vi "Add Network Chassis.vi"(0 "SLSC Remote in":refnum<class "SLSC Remote.lvclass">, 1 "username":string, 2 "password":string, 5 "chassis IP address/hostname":string, 11 "error in (no error)":errorcluster, 12 "connect timeout (60 sec)":dbl=60.0) -> (4 "SLSC Remote out":refnum<class "SLSC Remote.lvclass">, 6 "chassis out":refnum<k21>, 15 "error out":errorcluster)   [LabVIEW 2015, in "SLSC Remote.lvclass"]
uses:
  SLSC Remote.lvclass
  <vilib>/NI/i3 JSON/JSON Generation/Create Value Files/Create Value - Object.vi
  <vilib>/NI/i3 JSON/JSON Generation/Add Object Parameter Files/Add Object Parameter - String.vi
  <vilib>/NI/i3 JSON/JSON Generation/Add Object Parameter Files/Add Object Parameter - Numeric.vi
  <vilib>/NI/NI JSONRPC Server Framework/Classes/Server/Format Client Request (Auto-Increment).vi
  <vilib>/httpClient/POSTBuffer.vi
  <vilib>/NI/i3 JSON/JSON Parsing/Get Object Parameter Files/Get Object Parameter - String.vi
  <vilib>/NI/NI JSONRPC Server Framework/Classes/Server/JSONRPC Server.lvclass
  <vilib>/NI/i3 JSON/i3-json.lvlib
  <vilib>/httpClient/LabVIEWHTTPClient.lvlib
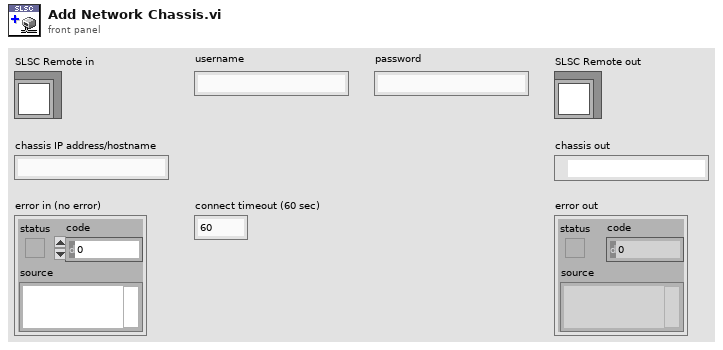
[diagram p1: front panel]
types:
  T1 = typedef "LabVIEWHTTPClient.lvlib/ClientHandle.ctl" = refnum<k1>
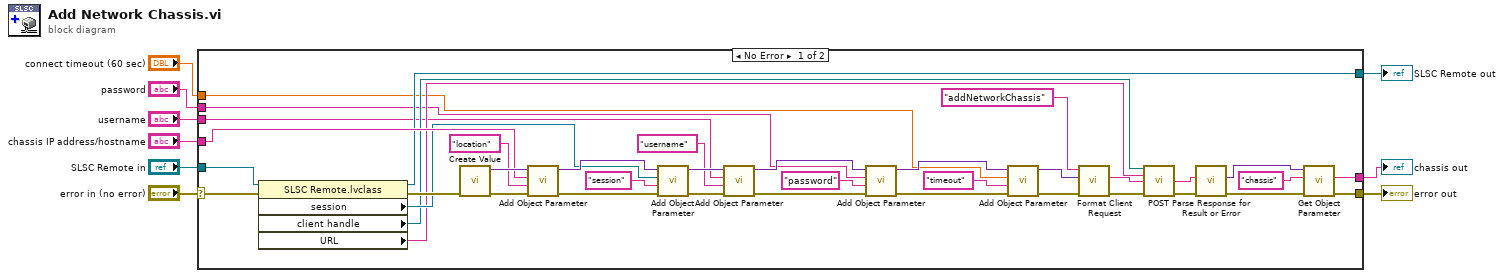
[diagram p0: block diagram]
diagram:
  n1 = case shown="No Error" "error in (no error)" {
    selector: "error in (no error)" -> [w42 w48]
    tunnel: "chassis IP address/hostname" -> [w46 _]
    tunnel: "SLSC Remote in" -> [w44 w49]
    tunnel: [w43 w49] -> w4
    tunnel: [w10 w48] -> w2
    tunnel: "username" -> [w23 _]
    tunnel: "password" -> [w21 _]
    tunnel: "connect timeout (60 sec)" -> [w17 _]
    tunnel: [w12 _] -> w3
    frame No Error {
      n2 = property class="SLSC Remote.lvclass"(reference=w44, error in=w42) -> (reference out=w43:refnum<class "SLSC Remote.lvclass">, error out=w41:errorcluster, "session"=w35:refnum<k21>, "client handle"=w33:T1, "URL"=w32:string)
      n3 = call-poly <vilib>:"Create Value.vi"("error in (no error)"=w41) -> ("error out"=w40:errorcluster, "JSON Tree"=w47:variant)  [unwired: 9 in]
      n4 = call-poly <vilib>:"Add Object Parameter.vi"("error in (no error)"=w40, "Name"="location", "String"=w46, "JSON Tree in (JSON Object)"=w47) -> ("error out"=w39:errorcluster, "JSON Tree out (JSON Object)"=w36:variant)  [unwired: 6 in]
      n5 = call-poly <vilib>:"Add Object Parameter.vi"("error in (no error)"=w39, "Name"="session", "String"=w35, "JSON Tree in (JSON Object)"=w36) -> ("error out"=w28:errorcluster, "JSON Tree out (JSON Object)"=w27:variant)  [unwired: 6 in]
      n6 = call-poly <vilib>:"Add Object Parameter.vi"("error in (no error)"=w28, "Name"="username" ("String"), "String"=w23, "JSON Tree in (JSON Object)"=w27) -> ("error out"=w26:errorcluster, "JSON Tree out (JSON Object)"=w25:variant)  [unwired: 6 in]
      n7 = call-poly <vilib>:"Add Object Parameter.vi"("error in (no error)"=w26, "Name"="password", "String"=w21, "JSON Tree in (JSON Object)"=w25) -> ("error out"=w20:errorcluster, "JSON Tree out (JSON Object)"=w19:variant)  [unwired: 6 in]
      n8 = call-poly <vilib>:"Add Object Parameter.vi"("error in (no error)"=w20, "Name"="timeout", "Numeric"=w17, "JSON Tree in (JSON Object)"=w19) -> ("error out"=w16:errorcluster, "JSON Tree out (JSON Object)"=w15:variant)  [unwired: 6 in]
      n9 = call-poly <vilib>:"Format Client Request.vi"("error in (no error)"=w16, "params"=w15, "method"="addNetworkChassis") -> ("error out"=w31:errorcluster, "Request String"=w37:string)  [unwired: 7 in]
      n10 = call-poly <vilib>:"POST.vi"("client handle"=w33, "url"=w32, "buffer"=w37, "error in (no error)"=w31) -> ("body"=w30:string, "error out"=w29:errorcluster)  [unwired: 8 in, 2 out]
      n11 = call <vilib>:"Parse Response for Result or Error.vi"("error in"=w29, "Response String In"=w30) -> ("error out"=w11:errorcluster, "Result or Error Data"=w14:variant)  [unwired: 7 in, 1 out]
      n12 = call-poly <vilib>:"Get Object Parameter.vi"("error in (no error)"=w11, "Parameter Name"="chassis", "JSON Tree In (JSON Object)"=w14) -> ("error out"=w10:errorcluster, "String Value"=w12:string)  [unwired: 5 in, 2 out]
    }
    frame Error {
    }
  }
  "error out" <- w2
  "SLSC Remote out" <- w4
  "chassis out" <- w3
